vi "_Yt12_GenericTest.vi"(11 "YTESTER测试数据":T1 caption="不要修改！") -> (3 "YTESTER结论":T2)   [LabVIEW 2017]
doc: "VIClassID=YT_SSTEPFLAG_SIMPLETEST\nVIDescription=对某个变量进行判断的简单测试"
uses:
  YtCommon.lvlibp/yt`Step StepBaseInput.ctl
  Step`s VIs/YYLLIdea/yylltestresult/yylltestresult basis.ctl
  YtCommon.lvlibp/yt`Step StepResult.ctl
  YtCommon.lvlibp/yt`Step TestData.ctl
  YtCommon.lvlibp/yt`Step System Queue.ctl
  YtCommon.lvlibp
panel:
  in  "YTESTER开放参数":T5={"YTESTER_BaseInput"={"isTest"=TRUE, "isSkip"=FALSE, "StepName"="通用简易解析测试", "OnPass"=enum."Next", "OnFail"=enum."Next", "ReTestNumber"=0.0}, "数据源什么类型？"=enum."String类型", "String数据源"="", "NUM数据源"=0.0, "Bool数据源"=FALSE, "Smart预处理"=[], "合格依据"=enum."强制合格", "StringLimit-A"="", "UpperLimit-B"=0.0, "LowLimit-C"=0.0, "unit"=""}
  # "简易通用解析测试步骤"
  # "YT_SSTEPFLAG_SIMPLETEST"
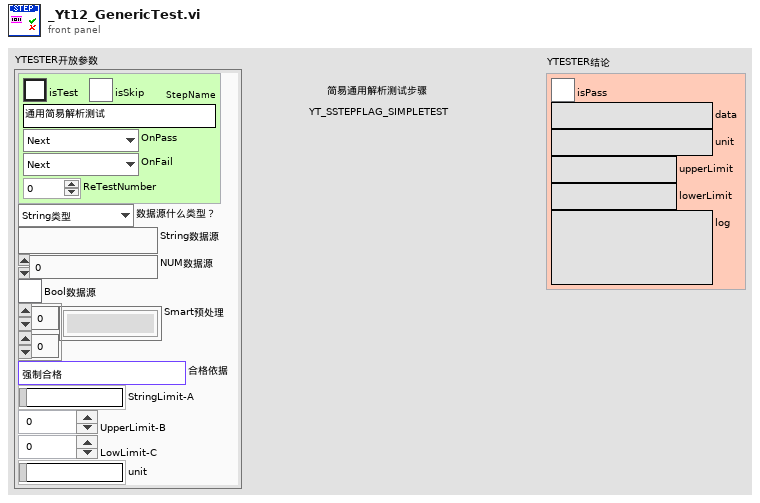
[diagram p1: front panel]
types:
  T1 = typedef "YtCommon.lvlibp/yt`Step TestData.ctl" = cluster{"Socket(From1)":i32, "SN":refnum<notifier>, "StopFlagRef":refnum<notifier>, "YT System Queue":refnum<queue>}
  T2 = typedef "YtCommon.lvlibp/yt`Step StepResult.ctl" = cluster{"isPass":bool, "data":string, "unit":string, "upperLimit":string, "lowerLimit":string, "log":string}
  T3 = typedef "YtCommon.lvlibp/yt`Step StepBaseInput.ctl" = cluster{"isTest":bool, "isSkip":bool, "StepName":string, "OnPass":enum16{"Next", "ToOVER", "Terminate"}, "OnFail":enum16{"Next", "ToOVER", "Terminate"}, "ReTestNumber":dbl}
  T4 = typedef "yylltestresult basis.ctl" = enum16{"强制合格", "强制不合格", "随机合格", "X=A", "X=\"真\"", "X=\"假\"", "X≠A", "X包含A", "X不包含A", "A包含X", "A包含非空X", "A不包含X", "X等于A正则匹配内容", "X包含A正则匹配内容", "X不包含A正则匹配内容", "X=B", "X≠B", "X＞B", "X≥B", "X＜B", "X≤B", "B≥X≥C", "B≥X＞C", "B＞X≥C", "B＞X＞C", "X≥B | C≥X", "X＞B | C≥X", "X≥B | C＞X", "X＞B | C＞X"}
  T5 = cluster{"YTESTER_BaseInput":T3, "数据源什么类型？":enum16{"String类型", "NUM类型", "Bool类型"}, "String数据源":string, "NUM数据源":dbl, "Bool数据源":bool, "Smart预处理":string[][], "合格依据":T4, "StringLimit-A":string, "UpperLimit-B":dbl, "LowLimit-C":dbl, "unit":string}
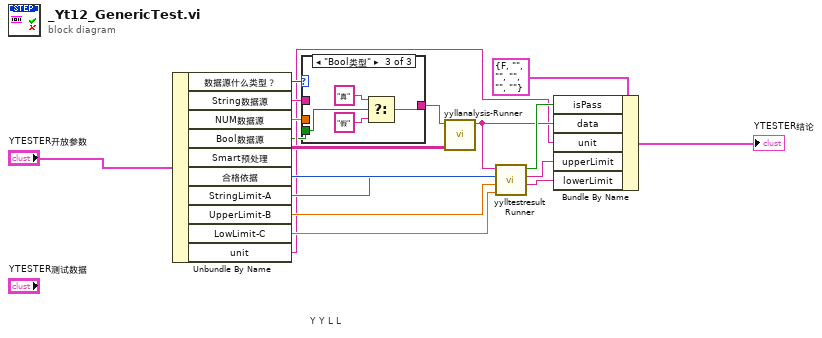
[diagram p0: block diagram]
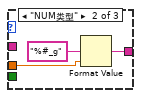
[diagram p3: hidden frame]
diagram:
  # "Y Y L L"
  n1 = Unbundle By Name("YTESTER开放参数") -> ("数据源什么类型？"=w15:enum16{"String类型", "NUM类型", "Bool类型"}, "String数据源"=w14:string, "NUM数据源"=w13:dbl, "Bool数据源"=w1:bool, "Smart预处理"=w11:string[][], "合格依据"=w10:T4, "StringLimit-A"=w9:string, "UpperLimit-B"=w8:dbl, "LowLimit-C"=w7:dbl, "unit"=w4:string)
  n2 = case shown="\"Bool类型\"" w15 {
    tunnel: w14 -> [w19 _ _]
    tunnel: [w19 w21 w24] -> w12
    tunnel: w13 -> [_ w22 _]
    tunnel: w1 -> [_ _ w23]
    frame "String类型" {
    }
    frame "NUM类型" {
      n3 = Format Value(format string="%#_g", value (0)=w22) -> (output string=w21:string)  [unwired: 1 in]
    }
    frame "Bool类型" {
      n4 = Select(t="真", s=w23, f="假") -> (s? t:f=w24:string)
    }
  }
  n5 = call "yyllanalysis-Runner.vi"("inputs"=w11, "String in"=w12) -> ("String out"=w5:string)  [unwired: 8 in, 1 out]
  n6 = call "yylltestresult Runner.vi"("合格依据"=w10, "LowLimit-C"=w7, "UpperLimit-B"=w8, "StringLimit-A"=w9, "DataIn-X"=w5) -> ("lowerLimit"=w2:string, "upperLimit"=w3:string, "isPass"=w6:bool)  [unwired: 4 in]
  n7 = Bundle By Name(cluster=T2 {"isPass"=FALSE, "data"="", "unit"="", "upperLimit"="", "lowerLimit"="", "log"=""} ("Result"), "isPass"=w6, "data"=w5, "unit"=w4, "upperLimit"=w3, "lowerLimit"=w2) -> (→"YTESTER结论":T2)
